vi "Save data to file.vi"(4 "DBC file name":string, 6 "Captured Data":string[][](array[string]), 7 "SAVE FORMAT":u16, 8 "error in":errorcluster, 9 "Headers":string[](array[string]), 10 "Bus Type":string, 11 "Path":path) -> (0 "error out":errorcluster, 3 "message":string)   [LabVIEW 2025, in "CAN-LIN Raw Bus Capture UI.lvlib"]
uses:
  CAN-LIN Raw Bus Capture UI.lvlib
  <vilib>/Utility/file.llb/Write Delimited Spreadsheet (string).vi
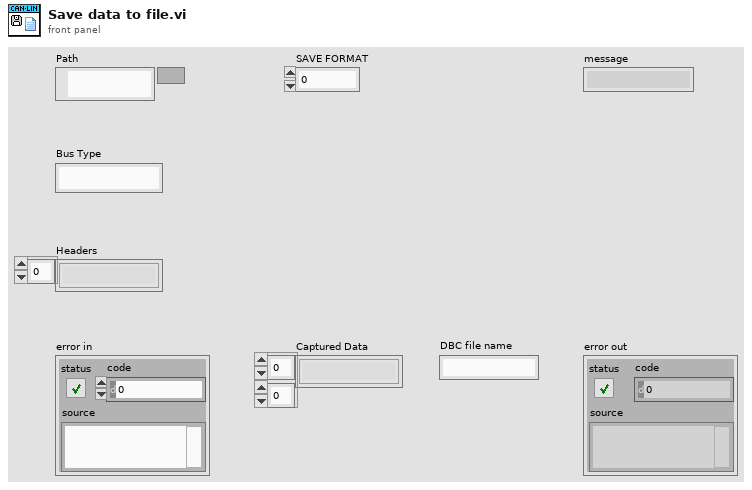
[diagram p1: front panel]
types:
  T1 = enum16{"open", "open or create", "create or replace", "create", "open (read-only)"}
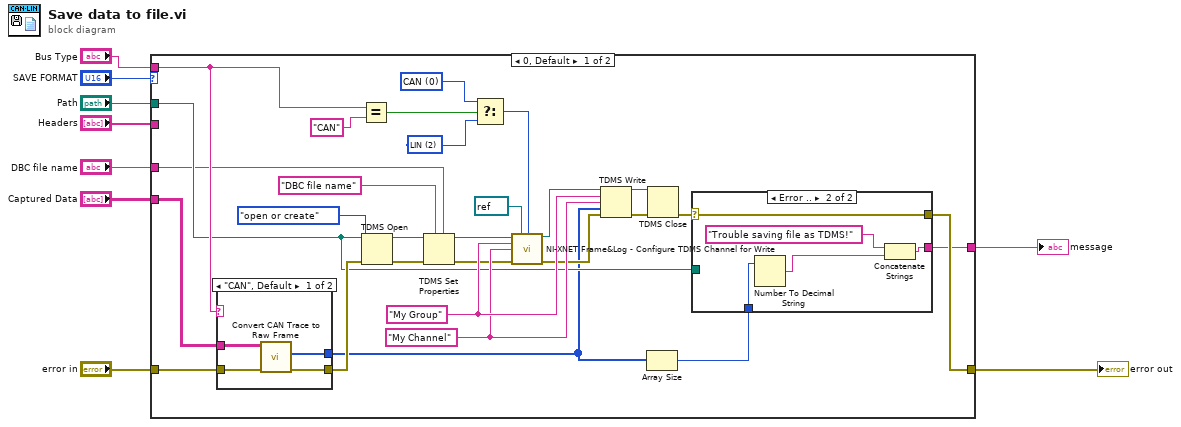
[diagram p0: block diagram]
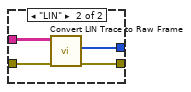
[diagram p2: hidden frame]
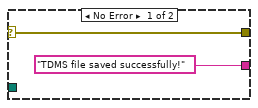
[diagram p3: hidden frame]
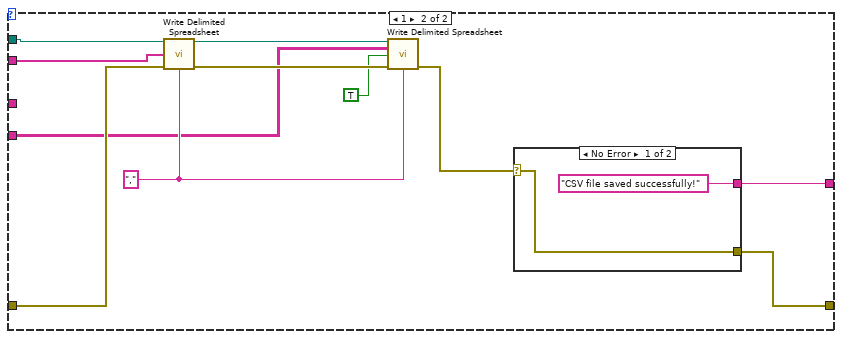
[diagram p4: hidden frame]
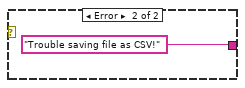
[diagram p5: hidden frame]
diagram:
  n1 = case shown="0, Default" "SAVE FORMAT" {
    tunnel: "Path" -> [w18 w60]
    tunnel: "Headers" -> [_ w59]
    tunnel: "error in" -> [w27 w58]
    tunnel: "Captured Data" -> [w28 w57]
    tunnel: [w32 w54] -> w5
    tunnel: [w31 w56] -> w7
    tunnel: "Bus Type" -> [w19 _]
    tunnel: "DBC file name" -> [w11 _]
    frame 0, Default {
      w30 = u32 0 items=["CAN", "FlexRay", "LIN"] ("protocol (CAN)")
      w23 = "My Channel" ("channel name")
      w24 = "My Group" ("group name (Untitled)")
      w29 = u32 2 items=["CAN", "FlexRay", "LIN"] ("protocol (CAN)")
      n2 = case shown="\"CAN\", Default" w19 {
        tunnel: w28 -> [w42 w46]
        tunnel: w27 -> [w41 w45]
        tunnel: [w40 w44] -> w26
        tunnel: [w39 w43] -> w17
        frame "CAN", Default {
          n3 = call "Convert CAN Trace to Raw Frame.vi"("error in"=w41, "captured data in"=w42) -> ("error out"=w40:errorcluster, "raw frames"=w39:u8[])  [unwired: 8 in]
        }
        frame "LIN" {
          n4 = call "Convert LIN Trace to Raw Frame.vi"("error in"=w45, "captured data in"=w46) -> ("error out"=w44:errorcluster, "raw frames"=w43:u8[])  [unwired: 8 in]
        }
      }
      n5 = Equal?(x=w19, y="CAN") -> (x = y?=w37:bool)
      n6 = TDMS Open(8:w26, 10:T1."open or create" ("operation (0:open)"), 11:w18) -> (0:w15:errorcluster, 3:w13:refnum<k34>)  [unwired: 4 in]
      n7 = TDMS Set Properties(5:w11, 7:"DBC file name" ("property names"), 8:w15, 11:w13) -> (0:w14:errorcluster, 3:w12:refnum<k34>)  [unwired: 2 in, 2 out]
      n8 = Select(t=w30, s=w37, f=w29) -> (s? t:f=w21:u32)
      n9 = call "NI-XNET Frame&Log - Configure TDMS Channel for Write.vi"("tdms file in"=w12, "XNET cluster (none)"=refnum<k21> refnum, "protocol (CAN)"=w21, "group name (Untitled)"=w24, "channel name"=w23, "error in (no error)"=w14) -> ("tdms file out"=w22:refnum<k34>, "error out"=w20:errorcluster)  [unwired: 7 in, 1 out]
      n10 = TDMS Write(0:w22, 5:w24, 7:w23, 9:w17, 11:w20) -> (4:w34:refnum<k34>, 15:w35:errorcluster)  [unwired: 1 in, 2 out]
      n11 = Array Size(array=w17) -> (size(s)=w16:i32)
      n12 = TDMS Close(8:w35, 11:w34) -> (0:w33:errorcluster)  [unwired: 1 out]
      n13 = case shown="Error .." w33 {
        selector: w33 -> [w48 w51]
        tunnel: [w48 w51] -> w32
        tunnel: ["TDMS file saved successfully!" ("message") w52] -> w31
        tunnel: w18 -> [_ _]
        tunnel: w16 -> [_ w50]
        frame No Error {
        }
        frame Error {
          n14 = Number To Decimal String(number=w50) -> (decimal integer string=w49:string)  [unwired: 1 in]
          n15 = Concatenate Strings("Trouble saving file as TDMS!" ("message"), w49) -> (w52:string)
        }
      }
    }
    frame 1 {
      w61 = "," ("delimiter (\\t)")
      n16 = call-poly <vilib>:"Write Delimited Spreadsheet.vi"("file path (dialog if empty)"=w60, "1D data"=w59, "error in (no error)"=w58, "delimiter (\\t)"=w61) -> ("new file path (Not A Path if cancelled)"=w62:path, "error out"=w64:errorcluster)  [unwired: 10 in]
      n17 = call-poly <vilib>:"Write Delimited Spreadsheet.vi"("file path (dialog if empty)"=w62, "2D data"=w57, "append to file? (new file:F)"=TRUE, "error in (no error)"=w64, "delimiter (\\t)"=w61) -> ("error out"=w55:errorcluster)  [unwired: 9 in, 1 out]
      n18 = case shown="No Error" w55 {
        selector: w55 -> [w65 _]
        tunnel: ["CSV file saved successfully!" ("message") "Trouble saving file as CSV!" ("message")] -> w56
        tunnel: [w65 _] -> w54
        frame No Error {
        }
        frame Error {
        }
      }
    }
  }
  "message" <- w7
  "error out" <- w5
